vi "TrimSpaceCol.vi"(8 "error in (no error)":errorcluster caption="エラー入力（エラーなし）", 10 "Bool Array":bool[](array[boolean]), 11 "Str Array":string[](array[string])) -> (0 "error out":errorcluster caption="エラー出力", 3 "Array out":string[](array[string]))   [LabVIEW 2015]
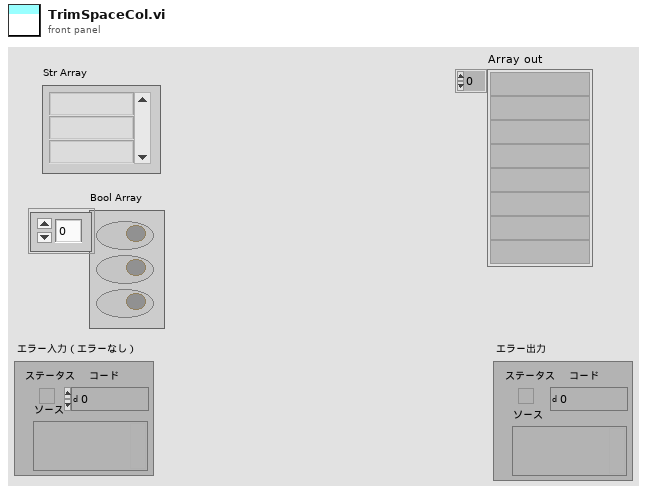
[diagram p1: front panel]
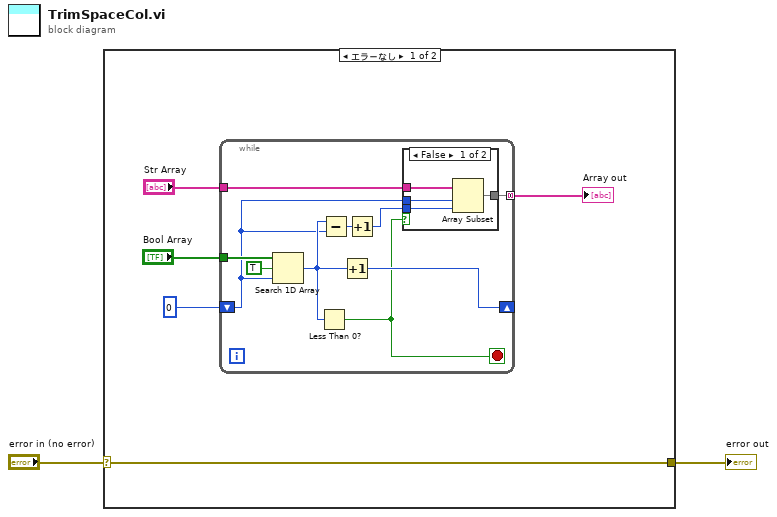
[diagram p0: block diagram]
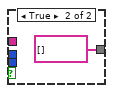
[diagram p2: hidden frame]
diagram:
  n1 = case shown="エラーなし" "error in (no error)" {
    selector: "error in (no error)" -> [w5 w23]
    tunnel: [w5 w23] -> w1
    frame No Error {
      n2 = while {
        tunnel: "Bool Array" -> [w17]
        shift-right: [w15] -> _
        shift-left: 0 -> [w12]
        tunnel: "Str Array" -> [w14]
        tunnel: [w11] -> w3 mode=concatenating
        stop <- w8 stop-if-true
        n3 = Search 1D Array(1D array=w17, element=TRUE ("要素"), start index (0)=w12) -> (index of element=w13:i32)
        n4 = Less Than 0?(x=w13) -> (x < 0?=w8:bool)
        n5 = Subtract(x=w13, y=w12) -> (x-y=w10:i32)
        n6 = Increment(x=w13) -> (x+1=w15:i32)
        n7 = Increment(x=w10) -> (x+1=w9:i32)
        n8 = case shown="FALSE" w8 {
          tunnel: w14 -> [w21 _]
          tunnel: w12 -> [w20 _]
          tunnel: [w19 string[] []] -> w11
          tunnel: w9 -> [w18 _]
          frame False {
            n9 = Array Subset(array=w21, index=w20, length=w18) -> (w19:string[])
          }
          frame True {
          }
        }
      }
      "Array out" <- w3
    }
    frame Error {
    }
  }
  "error out" <- w1
